vi "Read User Destination Signal.vi"(0 "signal index":u16, 2 "shared":refnum<class "niUSRP Rx Core v1 FPGA.lvclass">=refnum) -> (6 "conditioned signal":bool)   [LabVIEW 2023, in "niUSRP Rx Core v1 FPGA.lvclass"]
doc: "this VI reads a UserDestination signal from Routing, which can be configured from the host (e.g. - /deviceAlias/UserDestination0 )."
uses:
  <instrlib>/niUSRP/Reference FPGA/Rx Core/niUSRP Rx Core v1 FPGA.lvclass
  <instrlib>/niVST/Reference FPGA/FPGA/Routing/v1/Base/niVST Routing (Base) v1 FPGA.lvclass
  <instrlib>/niVST/Reference FPGA/FPGA/niUSRP Rx Core v1 FPGA/niUSRP Rx Core v1 FPGA.lvclass
  <instrlib>/niVST/Reference FPGA/FPGA/Routing/v1/Base/Public/Typedefs/User Destination Signal.ctl
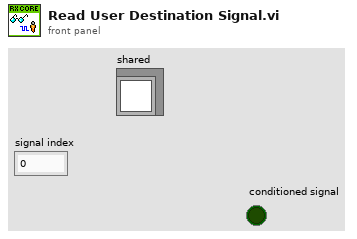
[diagram p1: front panel]
types:
  T1 = typedef "niVST Routing (Base) v1 FPGA.lvclass/User Destination Signal.ctl" = enum16{"UserDestination0", "UserDestination1", "UserDestination2", "UserDestination3", "UserDestination4", "UserDestination5", "UserDestination6", "UserDestination7"}
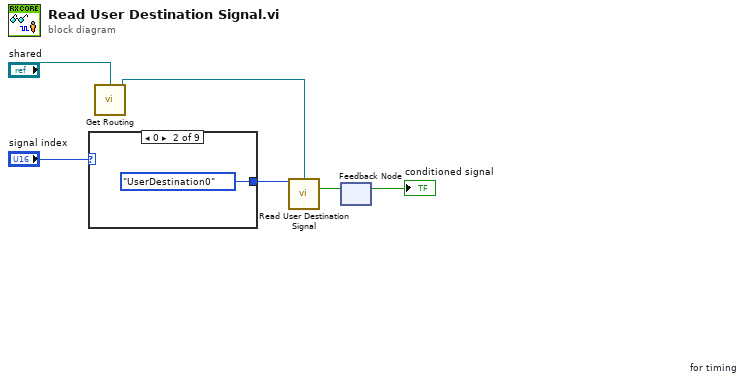
[diagram p0: block diagram]
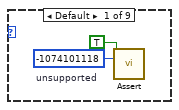
[diagram p2: hidden frame]
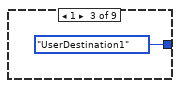
[diagram p3: hidden frame]
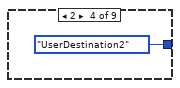
[diagram p4: hidden frame]
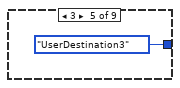
[diagram p5: hidden frame]
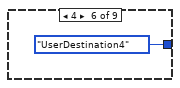
[diagram p6: hidden frame]
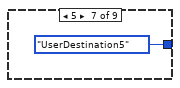
[diagram p7: hidden frame]
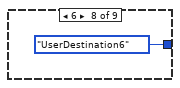
[diagram p8: hidden frame]
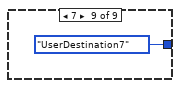
[diagram p9: hidden frame]
diagram:
  n1 = case shown="0" "signal index" {
    tunnel: [_ User_Destination_Signal."UserDestination0" ("signal select") User_Destination_Signal."UserDestination1" ("signal select") User_Destination_Signal."UserDestination2" ("signal select") User_Destination_Signal."UserDestination3" ("signal select") User_Destination_Signal."UserDestination4" ("signal select") User_Destination_Signal."UserDestination5" ("signal select") User_Destination_Signal."UserDestination6" ("signal select") User_Destination_Signal."UserDestination7" ("signal select")] -> w4
    frame Default {
      w7 = -1074101118  # unsupported
      n2 = call <instrlib>:"Assert.vi"("assert"=TRUE, "error code"=w7) -> ()  [unwired: 14 in]
    }
    frame 0 {
    }
    frame 1 {
    }
    frame 2 {
    }
    frame 3 {
    }
    frame 4 {
    }
    frame 5 {
    }
    frame 6 {
    }
    frame 7 {
    }
  }
  n3 = call-dynamic "Get Routing.vi"("shared"="shared") -> ("routing"=w3:refnum<class "niVST Routing (Base) v1 FPGA.lvclass">)  [unwired: 14 in]
  n4 = call-dynamic "Read User Destination Signal.vi"("signal select"=w4, "routing (Base)"=w3) -> ("conditioned signal"=w2:bool)  [unwired: 13 in]
  n5 = feedback-in #1(w2) -> ()
  n6 = feedback #1 "for timing"() -> (→"conditioned signal":bool)  [unwired: 1 in]
